vi "GetCursorPosition.vi"(8 "error in (no error)":errorcluster, 10 "DefaultHeight":i32, 11 "reference in":refnum<class "Row.lvclass">) -> (0 "error out":errorcluster, 1 "Dimensions":T1, 2 "CursorStartPoint":T2, 3 "reference in":refnum<class "Row.lvclass">)   [LabVIEW 2012, in "Row.lvclass"]
uses:
  Row.lvclass
  Glyph_class/Position.ctl
  Glyph_class/Dimensions.ctl
  Glyph_class/Glyph.lvclass
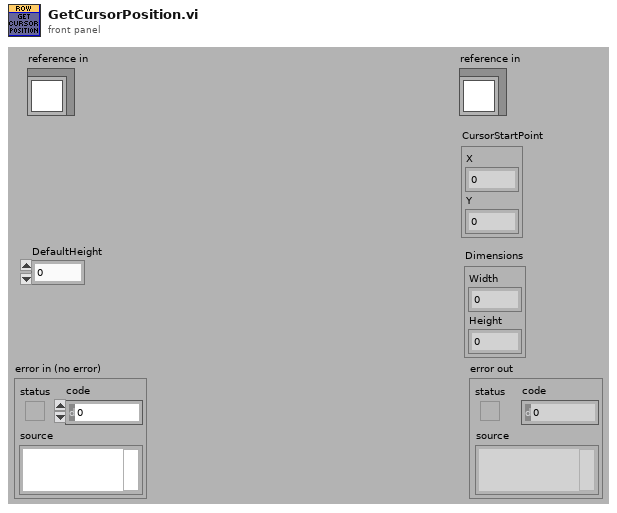
[diagram p1: front panel]
types:
  T1 = typedef "Glyph.lvclass/Dimensions.ctl" = cluster{"Width":i32, "Height":i32}
  T2 = typedef "Glyph.lvclass/Position.ctl" = cluster{"X":i32, "Y":i32}
  T3 = typedef "Row.lvclass/ObjectAttributes.ctl" = cluster{"Characters":refnum<class "Character.lvclass">[], "StartPoint":T2, "CharacterSpacing":i32}
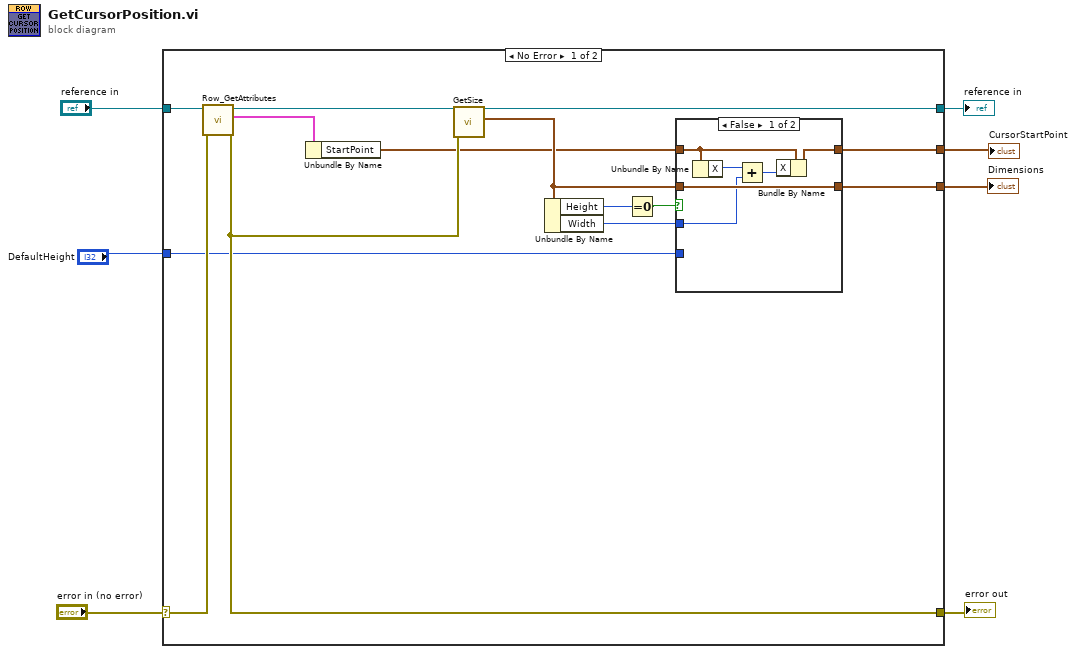
[diagram p0: block diagram]
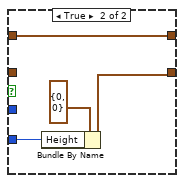
[diagram p2: hidden frame]
diagram:
  n1 = case shown="No Error" "error in (no error)" {
    selector: "error in (no error)" -> [w21 w33]
    tunnel: [w16 w33] -> w6
    tunnel: [w17 w32] -> w4
    tunnel: "reference in" -> [w19 w32]
    tunnel: [w9 _] -> w3
    tunnel: [w12 _] -> w2
    tunnel: "DefaultHeight" -> [w11 _]
    frame No Error {
      n2 = call "Row_GetAttributes.vi"("error in (no error)"=w21, "reference in"=w19) -> ("error out"=w16:errorcluster, "Data"=w20:T3, "reference out"=w18:refnum<class "Row.lvclass">)  [unwired: 6 in, 1 out]
      n3 = Unbundle By Name(w20) -> ("StartPoint"=w10:T2)
      n4 = call-dynamic "GetSize.vi"("error in (no error)"=w16, "reference in"=w18) -> ("Dimensions"=w13:T1, "reference in"=w17:refnum<class "Row.lvclass">)  [unwired: 7 in, 1 out]
      n5 = Unbundle By Name(w13) -> ("Height"=w15:i32, "Width"=w8:i32)
      n6 = Equal To 0?(x=w15) -> (x = 0?=w14:bool)
      n7 = case shown="False" w14 {
        tunnel: w13 -> [w27 _]
        tunnel: [w27 w30] -> w12
        tunnel: w11 -> [_ w29]
        tunnel: w10 -> [w26 w28]
        tunnel: [w25 w28] -> w9
        tunnel: w8 -> [w23 _]
        frame False {
          n8 = Unbundle By Name(w26) -> ("X"=w24:i32)
          n9 = Add(x=w24, y=w23) -> (x+y=w22:i32)
          n10 = Bundle By Name(cluster=w26, "X"=w22) -> (w25:T2)
        }
        frame True {
          n11 = Bundle By Name(cluster=T1 {"Width"=0, "Height"=0} ("Dimensions"), "Height"=w29) -> (w30:T1)
        }
      }
    }
    frame Error {
    }
  }
  "error out" <- w6
  "reference in" <- w4
  "CursorStartPoint" <- w3
  "Dimensions" <- w2
